vi "GetNodeInfo.vi"(6 "ns":u16=2, 8 "error in (no error)":errorcluster, 9 "id as String":string, 11 "Client In":refnum<class "Client.lvclass">) -> (0 "error out":errorcluster, 1 "Node Info":string, 2 "ret":i32, 3 "Client out":refnum<class "Client.lvclass">)   [LabVIEW 2017, in "opcua.lvlib" / "Client.lvclass"]
uses:
  Client.lvclass
  Client.lvclass/Client.ctl
  opcua.lvlib
  opcua32.dll
panel:
  # "could be i=84\nor s=MyFolder"
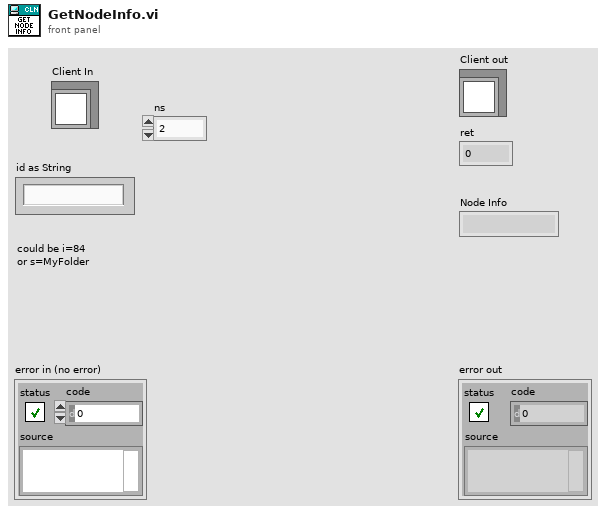
[diagram p1: front panel]
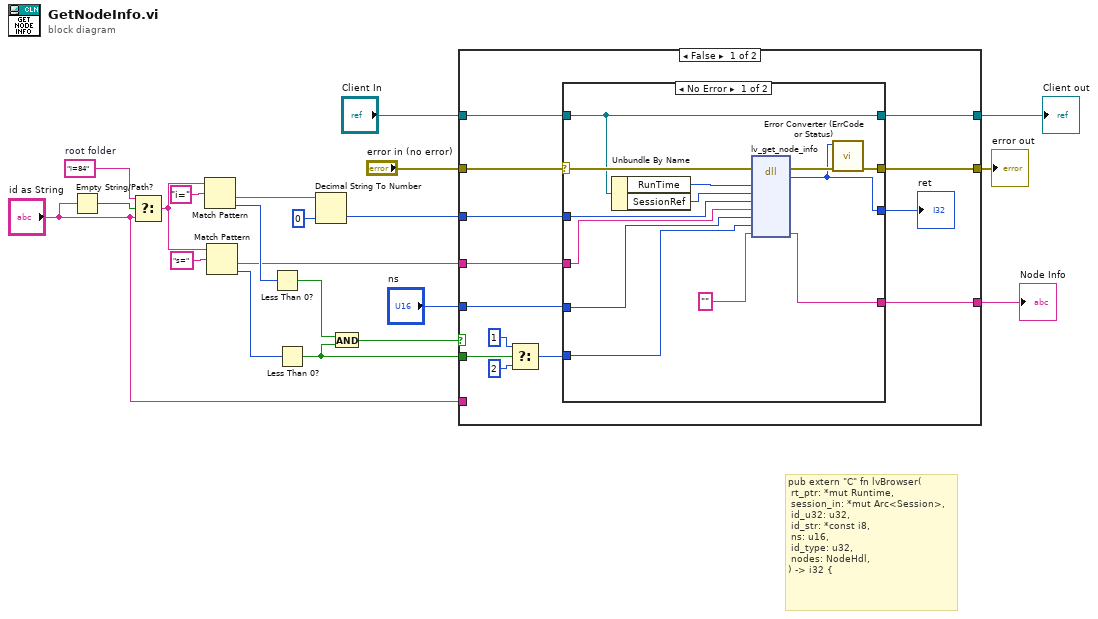
[diagram p0: block diagram]
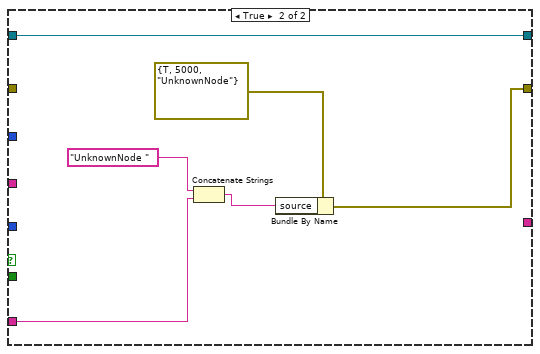
[diagram p3: hidden frame]
diagram:
  w4 = "i=84"  # root folder
  # "pub extern \"C\" fn lvBrowser(\n\trt_ptr: *mut Runtime,\n\tsession_in: *mut Arc<Session>,\n\tid_u32: u32,\n\tid_str: *const i8,\n\tns: u16,\n\tid_type: u32,\n\tnodes: NodeHdl,\n) -> i32 {"
  n1 = Empty String/Path?(string/path="id as String") -> (empty?=w5:bool)
  n2 = Select(t=w4, s=w5, f="id as String") -> (s? t:f=w3:string)
  n3 = Match Pattern(string=w3, regular expression="i=") -> (after substring=w13:string, offset past match=w12:i32)  [unwired: 1 in, 2 out]
  n4 = Match Pattern(string=w3, regular expression="s=") -> (after substring=w6:string, offset past match=w11:i32)  [unwired: 1 in, 2 out]
  n5 = Less Than 0?(x=w12) -> (x < 0?=w10:bool)
  n6 = Less Than 0?(x=w11) -> (x < 0?=w8:bool)
  n7 = Decimal String To Number(string=w13, default (0L)=u32 0 ("default (0 I32)")) -> (number=w15:u32)  [unwired: 1 in, 1 out]
  n8 = And(x=w10, y=w8) -> (x .and. y?=w9:bool)
  n9 = case shown="False" w9 {
    tunnel: "error in (no error)" -> [w34 _]
    tunnel: [w33 w50] -> w20
    tunnel: [w32 w55] -> w19
    tunnel: "Client In" -> [w31 w55]
    tunnel: w15 -> [w26 _]
    tunnel: w8 -> [w25 _]
    tunnel: w6 -> [w24 _]
    tunnel: "ns" -> [w23 _]
    tunnel: "id as String" -> [_ w52]
    tunnel: [w22 _] -> w1
    frame False {
      n10 = Select(t=1, s=w25, f=2) -> (s? t:f=w27:i32)
      n11 = case shown="No Error" w34 {
        selector: w34 -> [w46 w48]
        tunnel: [w39 w48] -> w33
        tunnel: [w44 w49] -> w32
        tunnel: w31 -> [w44 w49]
        tunnel: [w38 _] -> w30
        tunnel: w24 -> [w43 _]
        tunnel: w27 -> [w37 _]
        tunnel: w26 -> [w42 _]
        tunnel: w23 -> [w41 _]
        tunnel: [w35 _] -> w22
        frame No Error {
          n12 = Unbundle By Name(w44) -> ("RunTime"=w45:u64, "SessionRef"=w47:u64)
          n13 = dll-call lib="C:/Users/108003658/OneDrive - Baker Hughes/Desktop/opcua-0_2_0/opcua-lvlib/opcua*.dll" fn="lv_get_node_info"(error in=w46, "RunTime"=w45, "session"=w47, "id"=w42, "str"=w43, "ns"=w41, "type"=w37, "result"="") -> (error out=w40:errorcluster, "return type"=w38:i32, "result"=w35:string)  [unwired: 8 in, 1 out]
          n14 = call "Error Converter (ErrCode or Status).vi"("error in (no error)"=w40, "error code"=w38) -> ("error out"=w39:errorcluster)  [unwired: 9 in]
        }
        frame Error {
        }
      }
      "ret" <- w30
    }
    frame True {
      n15 = Concatenate Strings("UnknownNode " ("source"), w52) -> (w51:string)
      n16 = Bundle By Name(cluster=errorcluster {"status"=TRUE, "code"=5000, "source"="UnknownNode"} ("error IO"), "source"=w51) -> (w50:errorcluster)
    }
  }
  "error out" <- w20
  "Client out" <- w19
  "Node Info" <- w1
